vi "VFD.vi"() -> (0 "GS1 Communication Error Out":errorcluster)   [LabVIEW 2017]
uses:
  <vilib>/Platform/TimedLoop/XDataNode/timing_clust.ctl
  <vilib>/Platform/TimedLoop/XDataNode/nitl_modes.ctl
  <vilib>/Platform/TimedLoop/XDataNode/wakeup.ctl
  <vilib>/NI Modbus.llb/MB Serial Master Query Write Single Register (poly).vi
  <vilib>/Platform/TimedLoop/XDataNode/XDataNode.xnode
  <vilib>/Platform/TimedLoop/XDataNode/XDNodeRunTimeDep.lvlib
  <vilib>/NI Modbus.llb/MB Serial Master Query Read Holding Registers (poly).vi
panel:
  in  "GS1 Communication Error In":errorcluster
  out "Iteration Duration":i64
  out "Finished Late? [i-1]":bool
  out "TCHX Initializaton Error":errorcluster
  out "TCHX Initialization Loop Time (ms)":u32
  out "CTAH Initializaton Error":errorcluster
  out "CTAH Initialization Loop Time (ms)":u32
  out "Pump Initializaton Error":errorcluster
  out "Pump Initialization Loop Time (ms)":u32
  in  "Starting Address":u16
  out "Holding Registers":u16[](array[numeric])
  out "error out":errorcluster
  out "VISA resource name out":refnum<visa-resource-name>
  out "400001":u16
  out "error out":errorcluster
  # "Troubleshooting Modbus communication using third-party VIs and native I/O Server"
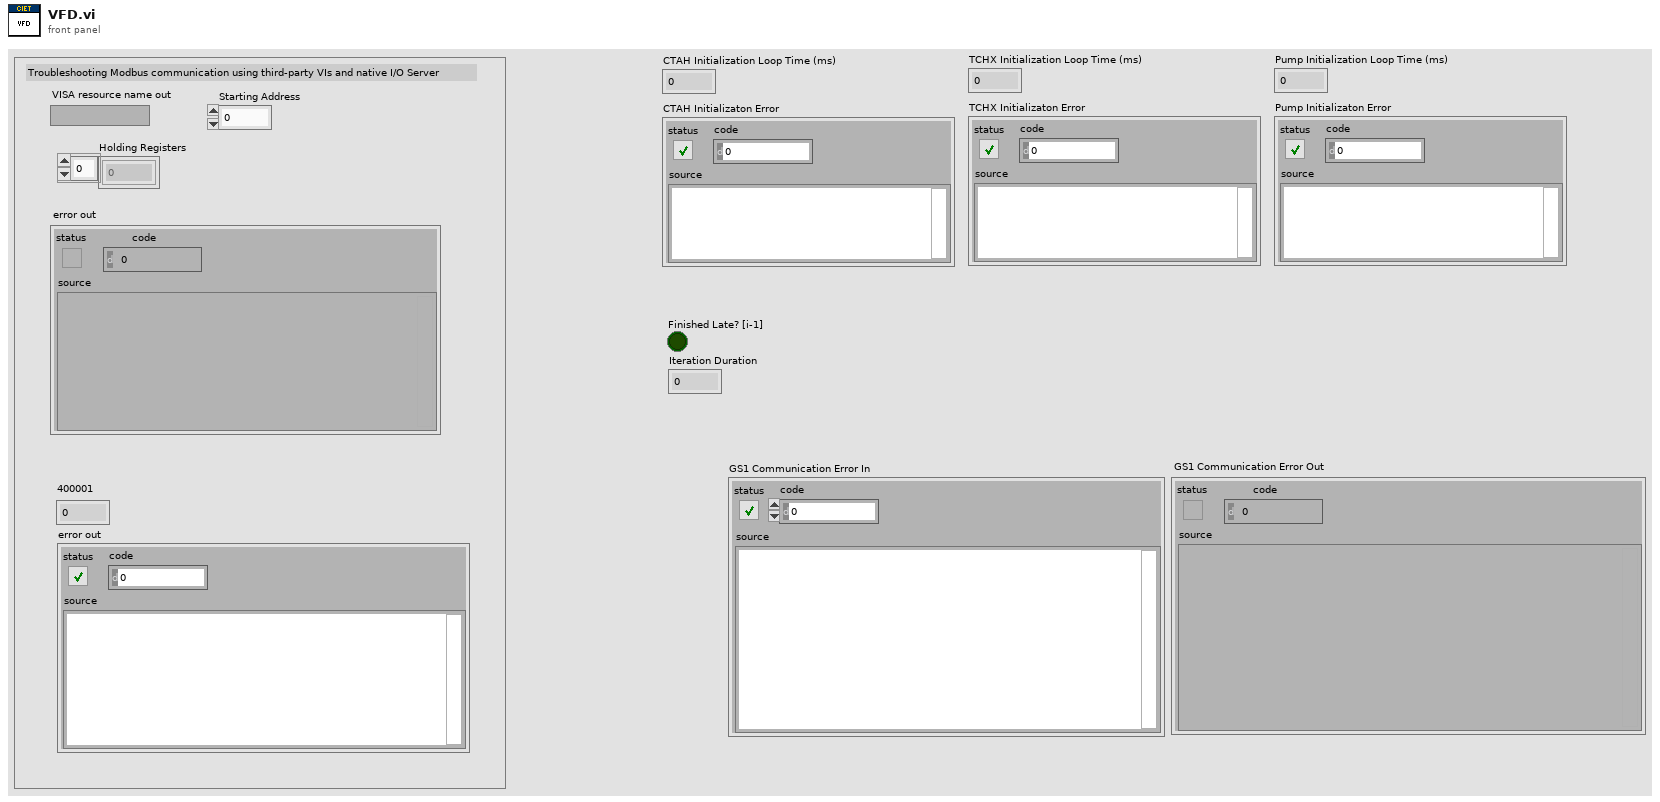
[diagram p1: front panel]
types:
  T1 = cluster{"Mode":enum16{"RTU", "ASCII"}, "Slave Address":u8}
  T2 = typedef "XDNodeRunTimeDep.lvlib/timing_clust.ctl" = cluster{"Expected End [f-1]":u64, "Actual End [f-1]":u64, "Finished Late? [f-1]":bool, "Expected End [i-1]":u64, "Actual End [i-1]":u64, "Finished Late? [i-1]":bool, "Expected Start [i]":u64, "Actual Start [i]":u64, "Expected Start [f]":u64, "Actual Start [f]":u64, "Source Name":string, "Structure Name":string, "Period":i64, "Deadline":i64, "Offset":i64, "Start":i64, "Priority":i32, "Timeout":i32, "Mode":T3, "Wakeup Reason":T4, "Error":errorcluster, "Source Type":string, "Secondary Source Type":string, "Global End Time":u64, "Global Start Time":u64, "Frame Duration":u64, "Iteration Duration":u64, "Assigned CPU":i32, "I/O Scan Engine Mode":u32}
  T3 = typedef "XDNodeRunTimeDep.lvlib/nitl_modes.ctl" = enum32{"No Change", "Process missed periods, maintain original phase", "Discard missed periods, maintain original phase", "Process missed periods, ignore original phase", "Discard missed periods, ignore original phase"}
  T4 = typedef "XDNodeRunTimeDep.lvlib/wakeup.ctl" = enum32{"Normal", "Aborted", "Asynchronous wakeup", "Timing source error", "Timed loop error", "Timeout"}
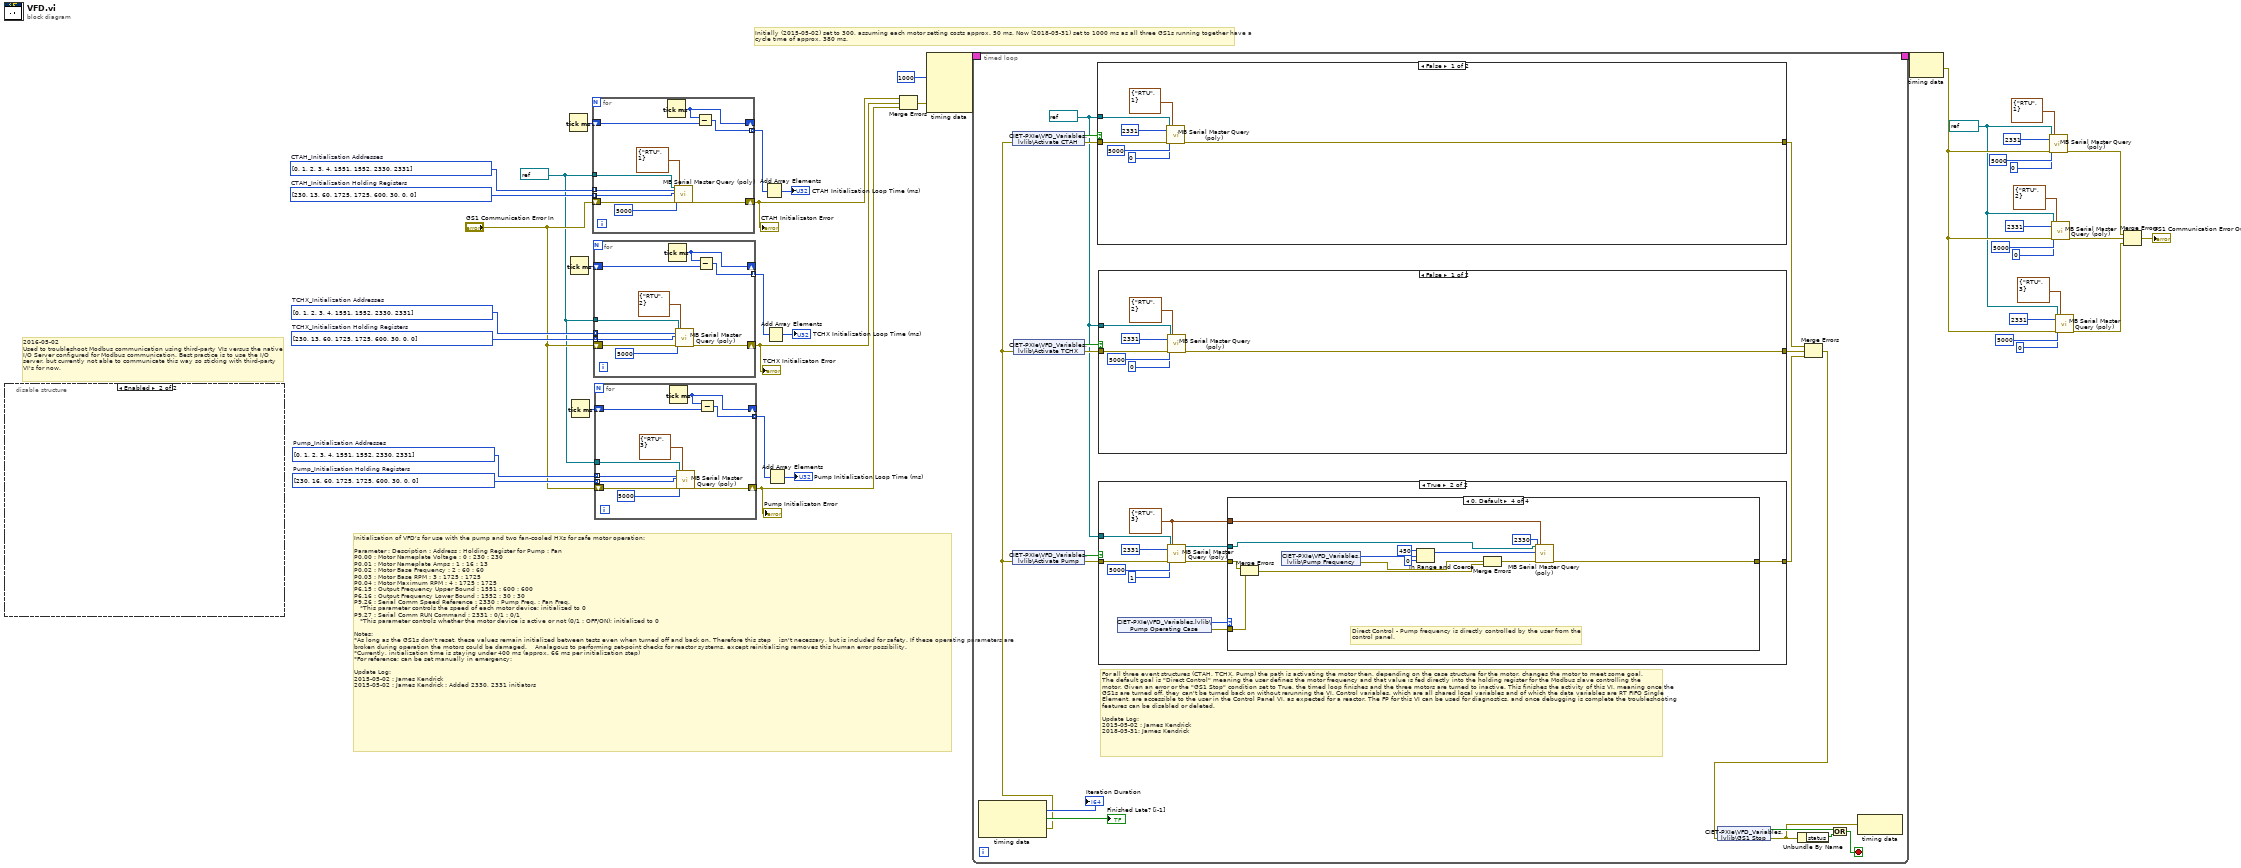
[diagram p0: block diagram]
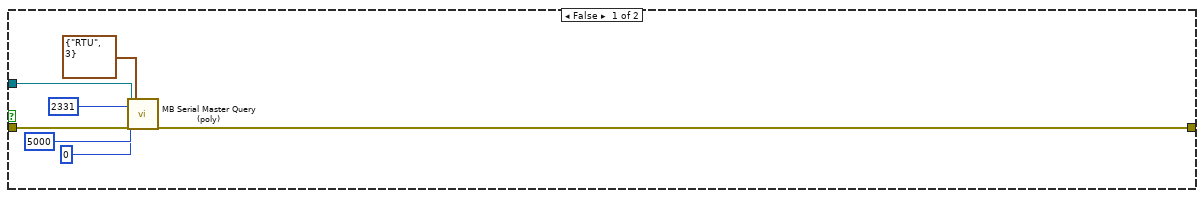
[diagram p2: hidden frame]
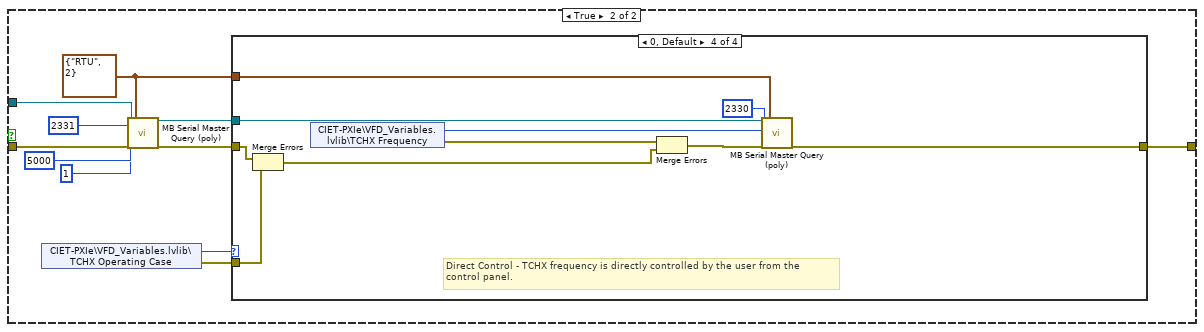
[diagram p6: hidden frame]
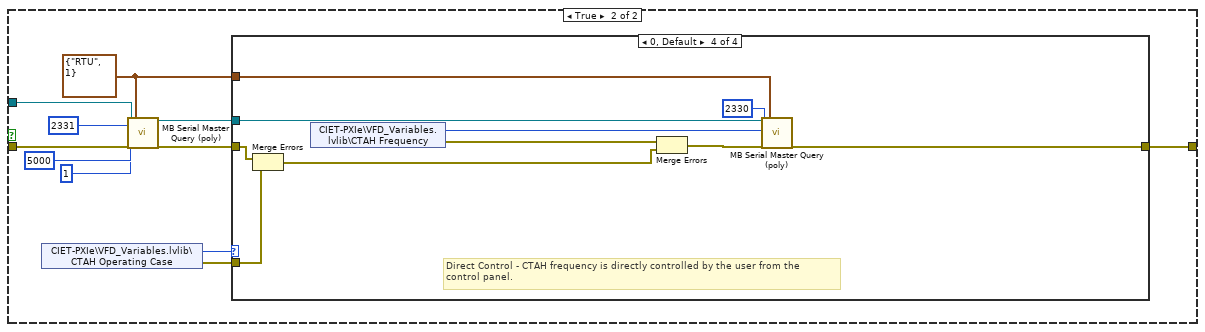
[diagram p10: hidden frame]
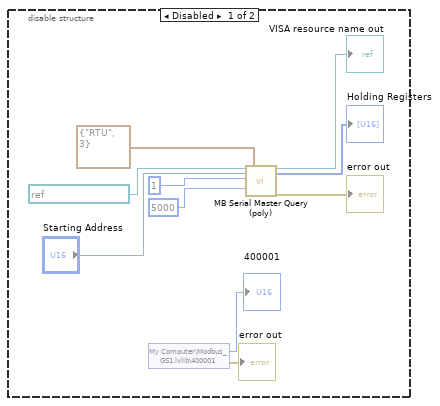
[diagram p14: hidden frame]
diagram:
  w4 = refnum<visa-resource-name> "VFD" ("VISA resource name")
  w5 = refnum<visa-resource-name> "VFD" ("VISA resource name")
  w28 = u16[] [230, 13, 60, 1725, 1725, 600, 30, 0, 0]  # TCHX_Initialization Holding Registers
  w29 = u16[] [0, 1, 2, 3, 4, 1551, 1552, 2330, 2331]  # TCHX_Initialization Addresses
  w33 = u16[] [230, 13, 60, 1725, 1725, 600, 30, 0, 0]  # CTAH_Initialization Holding Registers
  w34 = u16[] [0, 1, 2, 3, 4, 1551, 1552, 2330, 2331]  # CTAH_Initialization Addresses
  w41 = u16[] [230, 16, 60, 1725, 1725, 600, 30, 0, 0]  # Pump_Initialization Holding Registers
  w42 = u16[] [0, 1, 2, 3, 4, 1551, 1552, 2330, 2331]  # Pump_Initialization Addresses
  # "Initially (2015-05-02) set to 300, assuming each motor setting costs approx. 50 ms. Now (2018-05-31) set to 1000 ms as all three GS1s running together have a \ncycle time of approx. 380 ms."
  # "2016-05-02\nUsed to troubleshoot Modbus communication using third-party VIs versus the native\nI/O Server configured for Modbus communication. Best practice is to use the I/O \nserver, but currently not able to communicate this way so sticking with third-party \nVI's for now."
  # "Initialization of VFD's for use with the pump and two fan-cooled HXs for safe motor operation:\n\nParameter : Description : Address : Holding Register for Pump : Fan\nP0.00 : Motor Nameplate Voltage : 0 : 230 : 230\nP0.01 : Motor Nameplate Amps : 1 : 16 : 13\nP0.02 : Motor Base Frequency : 2 : 60 : 60\nP0.03 : Motor Base RPM : 3 : 1725 : 1725\nP0.04 : Motor Maximum RPM : 4 : 1725 : 1725\nP6.15 : Output Frequency Upper Bound : 1551 : 600 : 600\nP6.16 : Output Frequency Lower Bound : 1552 : 30 : 30\nP9.26 : Serial Comm Speed Reference : 2330 : Pump Freq. : Fan Freq. \n   *This parameter controls the speed of each motor device; initialized to 0\nP9.27 : Serial Comm RUN Command : 2331 : 0/1 : 0/1\n   *This parameter controls whether the motor device is active or not (0/1 : OFF/ON); initialized to 0\n\nNotes:\n*As long as the GS1s don't reset, these values remain initialized between tests even when turned off and back on. Therefore this step    isn't necessary, but is included for safety. If these operating parameters are broken during operation the motors could be damaged.    Analagous to performing set-point checks for reactor systems, except reinitializing removes this human error possibility.\n*Currently, initialization time is staying under 400 ms (approx. 66 ms per initialization step)\n*For reference; can be set manually in emergency:\n\nUpdate Log:\n2015-05-02 : James Kendrick \n2015-05-02 : James Kendrick : Added 2330, 2331 initiators"
  n1 = disable-structure shown="Enabled" {
    frame Disabled {
      n2 = shared-variable "My Computer\\Modbus_GS1.lvlib\\400001"() -> (→"400001":u16, error out=→"error out":errorcluster)  [unwired: 1 in]
      n3 = call-poly <vilib>:"MB Serial Master Query (poly).vi"("VISA resource name"=refnum<visa-resource-name> "GS1_AC_Drive", "Starting Address"="Starting Address", "Quantity"=u16 1, "Timeout"=u32 5000, "Serial Parameters"=T1 {"Mode"=enum."RTU", "Slave Address"=3}) -> ("VISA resource name out"=→"VISA resource name out":refnum<visa-resource-name>, "Holding Registers"=→"Holding Registers":u16[], "error out"=→"error out":errorcluster)  [unwired: 11 in, 1 out]
    }
    frame Enabled {
    }
  }
  n4 = Tick Count (ms)() -> (millisecond timer value=w32:u32)
  n5 = Tick Count (ms)() -> (millisecond timer value=w27:u32)
  n6 = Tick Count (ms)() -> (millisecond timer value=w40:u32)
  n7 = for {
    shift-right: [w60] -> w13
    shift-left: "GS1 Communication Error In" -> [w61]
    tunnel: w34 -> [w59] mode=indexing
    tunnel: w33 -> [w58] mode=indexing
    shift-right: [w55] -> _
    shift-left: w32 -> [w57]
    tunnel: [w56] -> w31 mode=indexing
    tunnel: w5 -> [w54]
    n8 = Tick Count (ms)() -> (millisecond timer value=w55:u32)
    n9 = call-poly <vilib>:"MB Serial Master Query (poly).vi"("VISA resource name"=w54, "Address"=w59, "Holding Register"=w58, "Timeout"=u32 5000, "error in"=w61, "Serial Parameters"=T1 {"Mode"=enum."RTU", "Slave Address"=1}) -> ("error out"=w60:errorcluster)  [unwired: 11 in, 2 out]
    n10 = Subtract(x=w55, y=w57) -> (x-y=w56:u32)
  }
  "CTAH Initializaton Error" <- w13
  n11 = for {
    shift-right: [w70] -> w7
    shift-left: "GS1 Communication Error In" -> [w71]
    tunnel: w29 -> [w69] mode=indexing
    tunnel: w28 -> [w68] mode=indexing
    shift-right: [w65] -> _
    shift-left: w27 -> [w67]
    tunnel: [w66] -> w26 mode=indexing
    tunnel: w5 -> [w64]
    n12 = Tick Count (ms)() -> (millisecond timer value=w65:u32)
    n13 = call-poly <vilib>:"MB Serial Master Query (poly).vi"("VISA resource name"=w64, "Address"=w69, "Holding Register"=w68, "Timeout"=u32 5000, "error in"=w71, "Serial Parameters"=T1 {"Mode"=enum."RTU", "Slave Address"=2}) -> ("error out"=w70:errorcluster)  [unwired: 11 in, 2 out]
    n14 = Subtract(x=w65, y=w67) -> (x-y=w66:u32)
  }
  "TCHX Initializaton Error" <- w7
  n15 = for {
    shift-right: [w80] -> w6
    shift-left: "GS1 Communication Error In" -> [w81]
    tunnel: w42 -> [w79] mode=indexing
    tunnel: w41 -> [w78] mode=indexing
    shift-right: [w75] -> _
    shift-left: w40 -> [w77]
    tunnel: [w76] -> w39 mode=indexing
    tunnel: w5 -> [w74]
    n16 = Tick Count (ms)() -> (millisecond timer value=w75:u32)
    n17 = call-poly <vilib>:"MB Serial Master Query (poly).vi"("VISA resource name"=w74, "Address"=w79, "Holding Register"=w78, "Timeout"=u32 5000, "error in"=w81, "Serial Parameters"=T1 {"Mode"=enum."RTU", "Slave Address"=3}) -> ("error out"=w80:errorcluster)  [unwired: 11 in, 2 out]
    n18 = Subtract(x=w75, y=w77) -> (x-y=w76:u32)
  }
  "Pump Initializaton Error" <- w6
  n19 = Add Array Elements(numeric array=w31) -> (sum=→"CTAH Initialization Loop Time (ms)":u32)
  n20 = Add Array Elements(numeric array=w26) -> (sum=→"TCHX Initialization Loop Time (ms)":u32)
  n21 = Add Array Elements(numeric array=w39) -> (sum=→"Pump Initialization Loop Time (ms)":u32)
  n22 = Merge Errors(w13, w7, w6) -> (w15:errorcluster)
  n23 = node-c288(i64 1000 ("Pump Control Period (ms)"), w15) -> (w37:T2)  [unwired: 3 in]
  n24 = timed-loop {
    timing: w37 -> [_]
    timing-out: [_] -> w36
    stop <- w96 stop-if-true
    w83 = refnum<visa-resource-name> "VFD" ("VISA resource name")
    # "For all three event structures (CTAH, TCHX, Pump) the path is activating the motor then, depending on the case structure for the motor, changes the motor to meet some goal. \nThe default goal is \"Direct Control\" meaning the user defines the motor frequency and that value is fed directly into the holding register for the Modbus slave controlling the \nmotor. Given an error or the \"GS1 Stop\" condition set to True, the timed loop finishes and the three motors are turned to inactive. This finishes the activity of this VI, meaning once the\nGS1s are turned off, they can't be turned back on without rerunning the VI. Control variables, which are all shared local variables and of which the data variables are RT FIFO Single\nElement, are accessible to the user in the Control Panel VI, as expected for a reactor. The FP for this VI can be used for diagnostics, and once debugging is complete the troubleshooting\nfeatures can be disabled or deleted.  \n\nUpdate Log:\n2015-05-02 : James Kendrick\n2018-05-31: James Kendrick"
    n25 = node-c288() -> (→"Iteration Duration":i64, →"Finished Late? [i-1]":bool, w89:errorcluster)  [unwired: 1 in]
    n26 = shared-variable "CIET-PXIe\\VFD_Variables.lvlib\\Activate CTAH"(error in=w89) -> (w100:bool, error out=w99:errorcluster)
    n27 = shared-variable "CIET-PXIe\\VFD_Variables.lvlib\\Activate Pump"(error in=w89) -> (w93:bool, error out=w92:errorcluster)
    n28 = shared-variable "CIET-PXIe\\VFD_Variables.lvlib\\Activate TCHX"(error in=w89) -> (w95:bool, error out=w94:errorcluster)
    n29 = case shown="False" w100 {
      tunnel: w99 -> [w163 w173]
      tunnel: [w162 w169] -> w87
      tunnel: w83 -> [w161 w168]
      frame False {
        n30 = call-poly <vilib>:"MB Serial Master Query (poly).vi"("VISA resource name"=w161, "Address"=u16 2331, "Holding Register"=u16 0, "Timeout"=u32 5000, "error in"=w163, "Serial Parameters"=T1 {"Mode"=enum."RTU", "Slave Address"=1}) -> ("error out"=w162:errorcluster)  [unwired: 11 in, 2 out]
      }
      frame True {
        w167 = T1 {"Mode"=enum."RTU", "Slave Address"=1} ("Serial Parameters")
        n31 = shared-variable "CIET-PXIe\\VFD_Variables.lvlib\\CTAH Operating Case"() -> (w171:i32, error out=w170:errorcluster)  [unwired: 1 in]
        n32 = call-poly <vilib>:"MB Serial Master Query (poly).vi"("VISA resource name"=w168, "Address"=u16 2331, "Holding Register"=u16 1, "Timeout"=u32 5000, "error in"=w173, "Serial Parameters"=w167) -> ("VISA resource name out"=w172:refnum<visa-resource-name>, "error out"=w174:errorcluster)  [unwired: 11 in, 1 out]
        n33 = case shown="0, Default" w171 {
          tunnel: w174 -> [_ _ _ w186]
          tunnel: w172 -> [_ _ _ w187]
          tunnel: w170 -> [_ _ _ w185]
          tunnel: [_ _ _ w179] -> w169
          tunnel: w167 -> [_ _ _ w178]
          frame 1 {
            # "CTAH Outlet Temp: Feedback - CTAH frequency is determined by a\ncontrol function to hold the outlet temperature of the CTAH \nconstant."
          }
          frame 2 {
            # "Load Following - CTAH frequency is controlled to make the CTAH heat removal power\nto equal a user specified value through satisfying the equation: m_dot*c_P*(T_in - T_out)"
          }
          frame 3 {
            # "Dynamic Forcing - CTAH frequency is defined by a waveform function to drive the \nCTAH frequency and thus mass flow rate in a dynamic pattern, such as a square wave,\nsine wave, or other function as defined by the user.\n\nUser inputs to include:\nCTAH frequency set point (used as signal offset)\nSignal amplitude\nSignal frequency\nSignal type: sine, square, others?"
          }
          frame 0, Default {
            # "Direct Control - CTAH frequency is directly controlled by the user from the\ncontrol panel."
            n34 = Merge Errors(w186, w185) -> (w180:errorcluster)
            n35 = shared-variable "CIET-PXIe\\VFD_Variables.lvlib\\CTAH Frequency"() -> (w183:u16, error out=w181:errorcluster)  [unwired: 1 in]
            n36 = Merge Errors(w181, w180) -> (w182:errorcluster)
            n37 = call-poly <vilib>:"MB Serial Master Query (poly).vi"("VISA resource name"=w187, "Address"=u16 2330, "Holding Register"=w183, "error in"=w182, "Serial Parameters"=w178) -> ("error out"=w179:errorcluster)  [unwired: 12 in, 2 out]
          }
        }
      }
    }
    n38 = case shown="False" w95 {
      tunnel: w94 -> [w135 w145]
      tunnel: [w134 w141] -> w85
      tunnel: w83 -> [w133 w140]
      frame False {
        n39 = call-poly <vilib>:"MB Serial Master Query (poly).vi"("VISA resource name"=w133, "Address"=u16 2331, "Holding Register"=u16 0, "Timeout"=u32 5000, "error in"=w135, "Serial Parameters"=T1 {"Mode"=enum."RTU", "Slave Address"=2}) -> ("error out"=w134:errorcluster)  [unwired: 11 in, 2 out]
      }
      frame True {
        w139 = T1 {"Mode"=enum."RTU", "Slave Address"=2} ("Serial Parameters")
        n40 = shared-variable "CIET-PXIe\\VFD_Variables.lvlib\\TCHX Operating Case"() -> (w143:i32, error out=w142:errorcluster)  [unwired: 1 in]
        n41 = call-poly <vilib>:"MB Serial Master Query (poly).vi"("VISA resource name"=w140, "Address"=u16 2331, "Holding Register"=u16 1, "Timeout"=u32 5000, "error in"=w145, "Serial Parameters"=w139) -> ("VISA resource name out"=w144:refnum<visa-resource-name>, "error out"=w146:errorcluster)  [unwired: 11 in, 1 out]
        n42 = case shown="0, Default" w143 {
          tunnel: w146 -> [_ _ _ w158]
          tunnel: w144 -> [_ _ _ w159]
          tunnel: w142 -> [_ _ _ w157]
          tunnel: [_ _ _ w151] -> w141
          tunnel: w139 -> [_ _ _ w150]
          frame 1 {
            # "TCHX Outlet Temp: Feedback - TCHX frequency is determined by a\ncontrol function to hold the outlet temperature of the TCHX \nconstant."
          }
          frame 2 {
            # "Freezing Event - TCHX frequency is adjust to simulate a freezing transient or freeze\nevent within the TCHX, compromising the heat transfer path from the core to\nenvironment during a transient without use of the pump/CTAH."
          }
          frame 3 {
            # "Dynamic Forcing - TCHX frequency is defined by a waveform function to drive the \nTCHX frequency and thus mass flow rate in a dynamic pattern, such as a square wave,\nsine wave, or other function as defined by the user.\n\nUser inputs to include:\nTCHX frequency set point (used as signal offset)\nSignal amplitude\nSignal frequency\nSignal type: sine, square, others?"
          }
          frame 0, Default {
            # "Direct Control - TCHX frequency is directly controlled by the user from the\ncontrol panel."
            n43 = Merge Errors(w158, w157) -> (w152:errorcluster)
            n44 = shared-variable "CIET-PXIe\\VFD_Variables.lvlib\\TCHX Frequency"() -> (w155:u16, error out=w153:errorcluster)  [unwired: 1 in]
            n45 = Merge Errors(w153, w152) -> (w154:errorcluster)
            n46 = call-poly <vilib>:"MB Serial Master Query (poly).vi"("VISA resource name"=w159, "Address"=u16 2330, "Holding Register"=w155, "error in"=w154, "Serial Parameters"=w150) -> ("error out"=w151:errorcluster)  [unwired: 12 in, 2 out]
          }
        }
      }
    }
    n47 = case shown="True" w93 {
      tunnel: w92 -> [w104 w114]
      tunnel: [w103 w110] -> w84
      tunnel: w83 -> [w102 w109]
      frame False {
        n48 = call-poly <vilib>:"MB Serial Master Query (poly).vi"("VISA resource name"=w102, "Address"=u16 2331, "Holding Register"=u16 0, "Timeout"=u32 5000, "error in"=w104, "Serial Parameters"=T1 {"Mode"=enum."RTU", "Slave Address"=3}) -> ("error out"=w103:errorcluster)  [unwired: 11 in, 2 out]
      }
      frame True {
        w108 = T1 {"Mode"=enum."RTU", "Slave Address"=3} ("Serial Parameters")
        n49 = shared-variable "CIET-PXIe\\VFD_Variables.lvlib\\Pump Operating Case"() -> (w112:i32, error out=w111:errorcluster)  [unwired: 1 in]
        n50 = call-poly <vilib>:"MB Serial Master Query (poly).vi"("VISA resource name"=w109, "Address"=u16 2331, "Holding Register"=u16 1, "Timeout"=u32 5000, "error in"=w114, "Serial Parameters"=w108) -> ("VISA resource name out"=w113:refnum<visa-resource-name>, "error out"=w115:errorcluster)  [unwired: 11 in, 1 out]
        n51 = case shown="0, Default" w112 {
          tunnel: w115 -> [_ _ _ w131]
          tunnel: w113 -> [_ _ _ w120]
          tunnel: w111 -> [_ _ _ w130]
          tunnel: [_ _ _ w126] -> w110
          tunnel: w108 -> [_ _ _ w119]
          frame 1 {
            # "Mass Flow Rate: Feedback - Pump frequency is controlled through \na closed feedback to match a specified mass flow rate defined by \nthe user on the control panel."
          }
          frame 2 {
            # "Mass Flow Rate: Ramp - Pump frequency is controlled through a control function that\ncontrols the rate of change of the mass flow rate that the user specifies on the control\npanel to match a user desired final mass flow rate."
          }
          frame 3 {
            # "Dynamic Forcing - Pump frequency is defined by a waveform function to drive the \npump frequency and thus mass flow rate in a dynamic pattern, such as a square wave,\nsine wave, or other function as defined by the user.\n\nUser inputs to include:\nPump frequency set point (used as signal offset)\nSignal amplitude\nSignal frequency\nSignal type: sine, square, others?"
          }
          frame 0, Default {
            # "Direct Control - Pump frequency is directly controlled by the user from the\ncontrol panel."
            n52 = Merge Errors(w131, w130) -> (w127:errorcluster)
            n53 = shared-variable "CIET-PXIe\\VFD_Variables.lvlib\\Pump Frequency"() -> (w123:u16, error out=w121:errorcluster)  [unwired: 1 in]
            n54 = In Range and Coerce(upper limit=u16 450, x=w123, lower limit=u16 0) -> (coerced(x)=w122:u16)  [unwired: 1 out]
            n55 = Merge Errors(w121, w127) -> (w128:errorcluster)
            n56 = call-poly <vilib>:"MB Serial Master Query (poly).vi"("VISA resource name"=w120, "Address"=u16 2330, "Holding Register"=w122, "error in"=w128, "Serial Parameters"=w119) -> ("error out"=w126:errorcluster)  [unwired: 12 in, 2 out]
          }
        }
      }
    }
    n57 = Merge Errors(w87, w85, w84) -> (w86:errorcluster)
    n58 = shared-variable "CIET-PXIe\\VFD_Variables.lvlib\\GS1 Stop"(error in=w86) -> (w91:bool, error out=w88:errorcluster)
    n59 = Unbundle By Name(w88) -> ("status"=w90:bool)
    n60 = Or(x=w91, y=w90) -> (x .or. y?=w96:bool)
    n61 = node-c288(w88) -> ()  [unwired: 1 out]
  }
  n62 = node-c288(w36) -> (w8:errorcluster)
  n63 = call-poly <vilib>:"MB Serial Master Query (poly).vi"("VISA resource name"=w4, "Address"=u16 2331, "Holding Register"=u16 0, "Timeout"=u32 5000, "error in"=w8, "Serial Parameters"=T1 {"Mode"=enum."RTU", "Slave Address"=1}) -> ("error out"=w10:errorcluster)  [unwired: 11 in, 2 out]
  n64 = call-poly <vilib>:"MB Serial Master Query (poly).vi"("VISA resource name"=w4, "Address"=u16 2331, "Holding Register"=u16 0, "Timeout"=u32 5000, "error in"=w8, "Serial Parameters"=T1 {"Mode"=enum."RTU", "Slave Address"=2}) -> ("error out"=w11:errorcluster)  [unwired: 11 in, 2 out]
  n65 = call-poly <vilib>:"MB Serial Master Query (poly).vi"("VISA resource name"=w4, "Address"=u16 2331, "Holding Register"=u16 0, "Timeout"=u32 5000, "error in"=w8, "Serial Parameters"=T1 {"Mode"=enum."RTU", "Slave Address"=3}) -> ("error out"=w9:errorcluster)  [unwired: 11 in, 2 out]
  n66 = Merge Errors(w10, w11, w9) -> (→"GS1 Communication Error Out":errorcluster)
